vi "Utility_Single ToggleVI.vi"(11 "Boolean in":bool) -> (3 "Boolean out":bool)   [LabVIEW 2017]
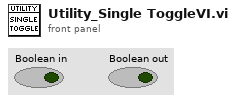
[diagram p1: front panel]
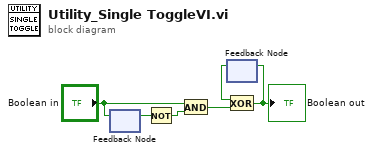
[diagram p0: block diagram]
diagram:
  n1 = feedback #1() -> (w1:bool)  [unwired: 1 in]
  n2 = feedback-in #1("Boolean in") -> ()
  n3 = Not(x=w1) -> (.not. x?=w2:bool)
  n4 = And(x="Boolean in", y=w2) -> (x .and. y?=w5:bool)
  n5 = feedback #2() -> (w4:bool)  [unwired: 1 in]
  n6 = Exclusive Or(1:w5, 2:w4) -> (0:w6:bool)
  "Boolean out" <- w6
  n7 = feedback-in #2(w6) -> ()
